vi "set_remote-interface-mode.vi"(8 "error in (no error)":errorcluster, 10 "mode":u16(ring) items=["local", "remote", "remot with lock-out"], 11 "LakeShore336 in":refnum<class "Lakeshore_336.lvclass">) -> (0 "error out":errorcluster, 3 "LakeShore336 out":refnum<class "Lakeshore_336.lvclass">)   [LabVIEW 2018, in "Lakeshore_336.lvclass"]
doc: "sets the remote interface of the actual instrument.\nMode=1 (local), 2 (remote), 3 (remote with lockout)"
uses:
  Lakeshore_336.lvclass
  instrument.lvclass
  Drivers/Lake Shore 336/Lake Shore 336.lvlib
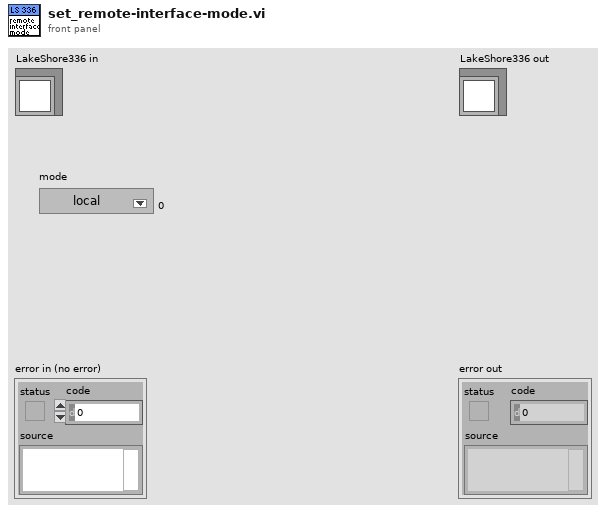
[diagram p1: front panel]
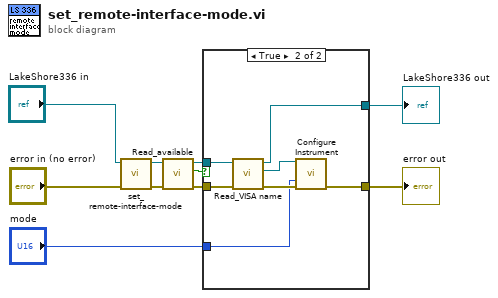
[diagram p0: block diagram]
diagram:
  n1 = call-parent "set_remote-interface-mode.vi"("error in (no error)"="error in (no error)", "instrument in"="LakeShore336 in") -> ("error out"=w4:errorcluster, "instrument out"=w5:refnum<class "Lakeshore_336.lvclass">)  [unwired: 8 in]
  n2 = call-dynamic "Read_available.vi"("error in (no error)"=w4, "instrument in"=w5) -> ("error out"=w2:errorcluster, "available?"=w1:bool, "instrument out"=w3:refnum<class "Lakeshore_336.lvclass">)  [unwired: 7 in]
  n3 = case shown="True" w1 {
    tunnel: [w12 w19] -> w8
    tunnel: "mode" -> [_ w16]
    tunnel: [w11 w15] -> w6
    tunnel: w3 -> [w12 w14]
    tunnel: w2 -> [w11 w13]
    frame False {
    }
    frame True {
      n4 = call-dynamic "Read_VISA name.vi"("error in (no error)"=w13, "instrument in"=w14) -> ("error out"=w18:errorcluster, "VISA resource name"=w17:refnum<visa-resource-name>, "instrument out"=w19:refnum<class "Lakeshore_336.lvclass">)  [unwired: 7 in]
      n5 = call "Configure Instrument.vi"("VISA resource name"=w17, "Remote Interface Mode (0:Local)"=w16, "error in (no error)"=w18) -> ("error out"=w15:errorcluster)  [unwired: 11 in, 1 out]
    }
  }
  "error out" <- w6
  "LakeShore336 out" <- w8
